vi "Move the pointer.vi"(2 "error in (no error)":errorcluster, 3 "Servo Angles":cluster{"Angle X":dbl, "Angle Y":dbl}, 4 "Device In":i32) -> (0 "error out":errorcluster, 1 "Device Out":i32)   [LabVIEW 2014]
doc: "This vi will move the servos to the angles passed in radians to position the pointer."
panel:
  out "Y servo":dbl
  out "X servo":dbl
  out "Y degrees":dbl
  out "X degrees":dbl
  in  "Y zero":dbl=145.0
  in  "Y Gain":dbl=0.91
  in  "X zero":dbl=112.0
  in  "X Gain":dbl=0.91
  in  "Y Offset":dbl
  in  "X Offset":dbl
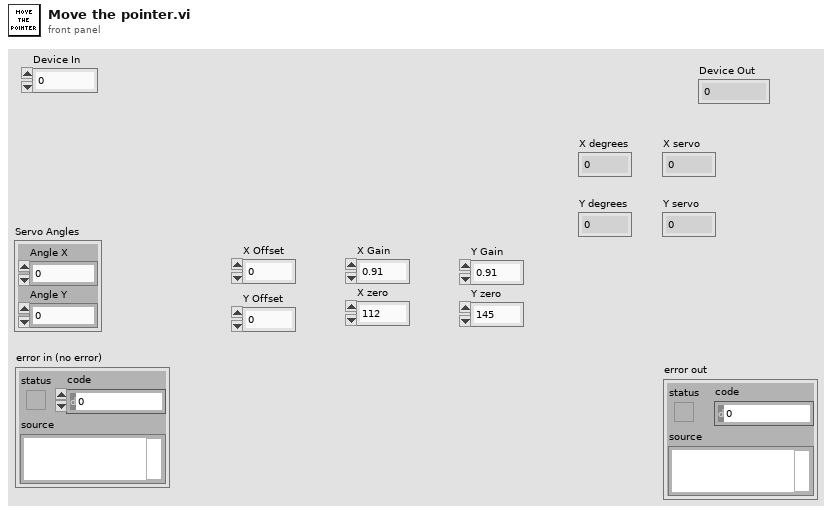
[diagram p1: front panel]
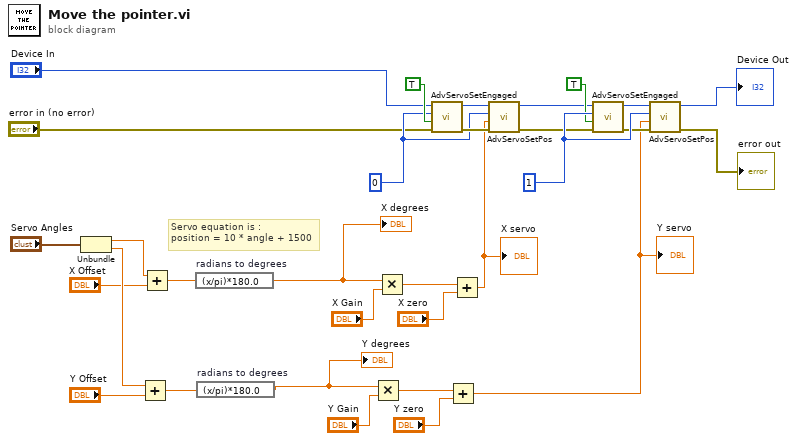
[diagram p0: block diagram]
diagram:
  w13 = 1
  w14 = 0
  # "Servo equation is :\nposition = 10 * angle + 1500"
  n1 = Unbundle("Servo Angles") -> ("Angle X"=w30:dbl, "Angle Y"=w29:dbl)
  n2 = Add(x=w29, y="Y Offset") -> (x+y=w26:dbl)
  n3 = Add(x=w30, y="X Offset") -> (x+y=w27:dbl)
  n4 = expression code="(x/pi)*180.0" "radians to degrees"(w27) -> (w25:dbl)
  "X degrees" <- w25
  n5 = expression code="(x/pi)*180.0" "radians to degrees"(w26) -> (w18:dbl)
  "Y degrees" <- w18
  n6 = Multiply(x=w18, y="Y Gain") -> (x*y=w20:dbl)
  n7 = Multiply(x=w25, y="X Gain") -> (x*y=w23:dbl)
  n8 = call "AdvServoSetEngaged.vi"("error in (no error)"="error in (no error)", "SetEngaged"=TRUE, "index"=w14, "Device In"="Device In") -> ("error out"=w15:errorcluster, "Device Out"=w16:i32)  [unwired: 5 in]
  n9 = Add(x=w20, y="Y zero") -> (x+y=w2:dbl)
  "Y servo" <- w2
  n10 = Add(x=w23, y="X zero") -> (x+y=w3:dbl)
  "X servo" <- w3
  n11 = call "AdvServoSetPos.vi"("error in (no error)"=w15, "pos_in"=w3, "index"=w14, "Device In"=w16) -> ("error out"=w8:errorcluster, "Device Out"=w9:i32)  [unwired: 5 in]
  n12 = call "AdvServoSetEngaged.vi"("error in (no error)"=w8, "SetEngaged"=TRUE, "index"=w13, "Device In"=w9) -> ("error out"=w12:errorcluster, "Device Out"=w11:i32)  [unwired: 5 in]
  n13 = call "AdvServoSetPos.vi"("error in (no error)"=w12, "pos_in"=w2, "index"=w13, "Device In"=w11) -> ("error out"=→"error out":errorcluster, "Device Out"=→"Device Out":i32)  [unwired: 5 in]
